vi "Stop TimerDRV.vi"(7 "Keep Time Source?":bool, 8 "error in (no error)":errorcluster, 11 "TimerDRV in":refnum<class "TimerDRV.lvclass">) -> (0 "error out":errorcluster, 3 "TimerDRV out":refnum<class "TimerDRV.lvclass">)   [LabVIEW 2019, in "TimingDRV Engine.lvlib" / "TimerDRV.lvclass"]
uses:
  TimerDRV.lvclass
  TimerDRV.lvclass/TimerDRV.ctl
  TypeDefs/Command Package.ctl
  TypeDefs/Command.ctl
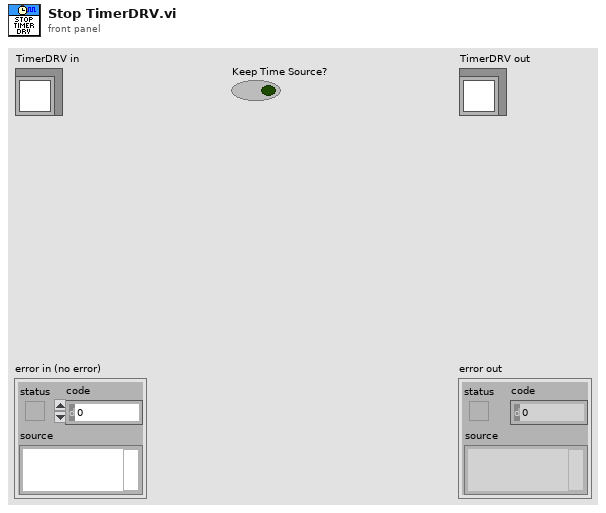
[diagram p1: front panel]
types:
  T1 = typedef "TimingDRV Engine.lvlib/TimerDRV.lvclass/Command Package.ctl" = cluster{"Command":T2, "Command Data":variant}
  T2 = typedef "TimingDRV Engine.lvlib/TimerDRV.lvclass/Command.ctl" = enum16{"Shutdown", "Update Execution Frequency", "Initialize"}
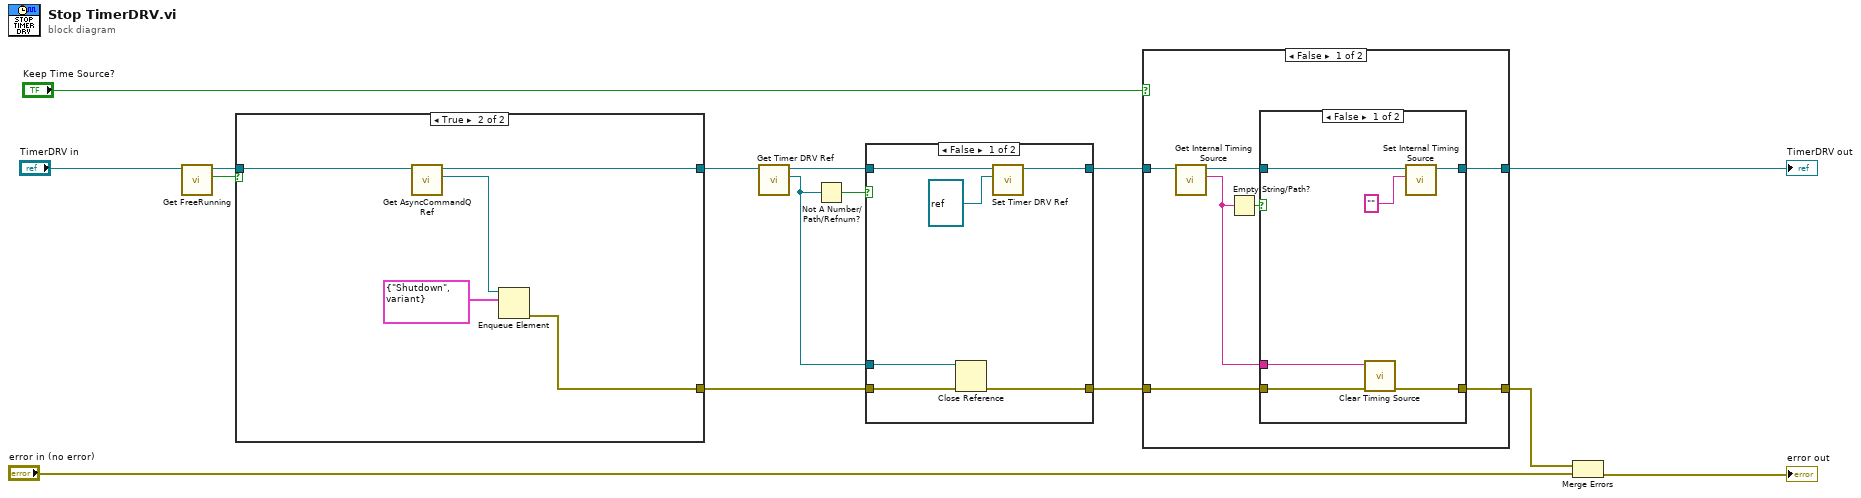
[diagram p0: block diagram]
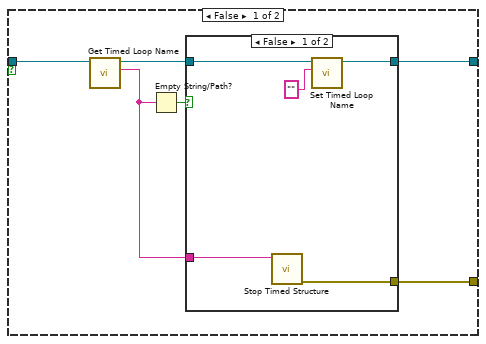
[diagram p2: hidden frame]
diagram:
  n1 = call "Get FreeRunning.vi"("TimerDRV in"="TimerDRV in") -> ("FreeRunning"=w5:bool, "TimerDRV out"=w4:refnum<class "TimerDRV.lvclass">)  [unwired: 9 in]
  n2 = case shown="True" w5 {
    tunnel: w4 -> [w18 w32]
    tunnel: [w16 w30] -> w3
    tunnel: [w17 w28] -> w2
    frame False {
      n3 = call "Get Timed Loop Name.vi"("TimerDRV in"=w18) -> ("Timed Loop Name"=w19:string, "TimerDRV out"=w21:refnum<class "TimerDRV.lvclass">)  [unwired: 9 in]
      n4 = Empty String/Path?(string/path=w19) -> (empty?=w20:bool)
      n5 = case shown="False" w20 {
        tunnel: w21 -> [w22 w27]
        tunnel: [w26 w27] -> w17
        tunnel: [w25 _] -> w16
        tunnel: w19 -> [w23 _]
        frame False {
          n6 = call <vilib>:"Stop Timed Structure.vi"("name"=w23) -> ("error out"=w25:errorcluster)  [unwired: 10 in]
          n7 = call "Set Timed Loop Name.vi"("Timed Loop Name"="", "TimerDRV in"=w22) -> ("TimerDRV out"=w26:refnum<class "TimerDRV.lvclass">)  [unwired: 9 in]
        }
        frame True {
        }
      }
    }
    frame True {
      n8 = call "Get AsyncCommandQ Ref.vi"("TimerDRV in"=w32) -> ("AsyncCommandQ"=w31:refnum<queue>, "TimerDRV out"=w28:refnum<class "TimerDRV.lvclass">)  [unwired: 9 in]
      n9 = Enqueue Element(queue=w31, element=T1 {"Command"=enum."Shutdown", "Command Data"=variant}) -> (error out=w30:errorcluster)  [unwired: 2 in, 2 out]
    }
  }
  n10 = call "Get Timer DRV Ref.vi"("TimerDRV in"=w2) -> ("Timer DRV Ref"=w8:refnum<vi>, "TimerDRV out"=w10:refnum<class "TimerDRV.lvclass">)  [unwired: 9 in]
  n11 = Not A Number/Path/Refnum?(number/path/refnum=w8) -> (NaN/Path/Refnum?=w9:bool)
  n12 = case shown="False" w9 {
    tunnel: w10 -> [w34 w40]
    tunnel: w3 -> [w38 w39]
    tunnel: [w37 w40] -> w7
    tunnel: [w36 w39] -> w15
    tunnel: w8 -> [w33 _]
    frame False {
      n13 = Close Reference(reference=w33, error in (no error)=w38) -> (error out=w36:errorcluster)
      n14 = call "Set Timer DRV Ref.vi"("Timer DRV Ref"=refnum<vi> refnum, "TimerDRV in"=w34) -> ("TimerDRV out"=w37:refnum<class "TimerDRV.lvclass">)  [unwired: 9 in]
    }
    frame True {
    }
  }
  n15 = case shown="False" "Keep Time Source?" {
    tunnel: w15 -> [w47 w56]
    tunnel: [w46 w56] -> w13
    tunnel: [w45 w57] -> w11
    tunnel: w7 -> [w43 w57]
    frame False {
      n16 = call "Get Internal Timing Source.vi"("TimerDRV in"=w43) -> ("Internal Timing Source"=w42:string, "TimerDRV out"=w44:refnum<class "TimerDRV.lvclass">)  [unwired: 9 in]
      n17 = Empty String/Path?(string/path=w42) -> (empty?=w41:bool)
      n18 = case shown="False" w41 {
        tunnel: [w53 w55] -> w46
        tunnel: [w52 w54] -> w45
        tunnel: w47 -> [w51 w55]
        tunnel: w42 -> [w49 _]
        tunnel: w44 -> [w48 w54]
        frame False {
          n19 = call <vilib>:"Clear Timing Source.vi"("error in (no error)"=w51, "name"=w49) -> ("error out"=w53:errorcluster)  [unwired: 8 in, 1 out]
          n20 = call "Set Internal Timing Source.vi"("Internal Timing Source"="" ("Timing Source"), "TimerDRV in"=w48) -> ("TimerDRV out"=w52:refnum<class "TimerDRV.lvclass">)  [unwired: 9 in]
        }
        frame True {
        }
      }
    }
    frame True {
    }
  }
  "TimerDRV out" <- w11
  n21 = Merge Errors(w13, "error in (no error)") -> (→"error out":errorcluster)
